vi "nanomsg_ctx_create.vi"(3 "error in":errorcluster) -> (0 "error out":errorcluster, 2 "context out":refnum<class "nanomsg_context.lvclass">)   [LabVIEW 2014, in "nanomsg.lvlib" / "nanomsg_context.lvclass"]
doc: "Instantiate Nanomsg and return a <b>context</b> to create sockets with. Ideally, this should only be called once per application and the context shared."
uses:
  nanomsg_context.lvclass
  nanomsg_context.lvclass/nanomsg_context.ctl
  <vilib>/Utility/error.llb/Error Cluster From Error Code.vi
  nanomsg.lvlib
panel:
  # "NN"
  # "labview"
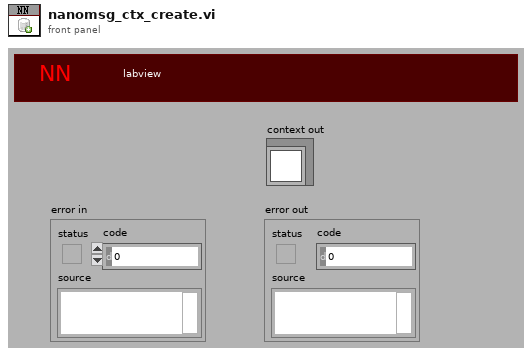
[diagram p1: front panel]
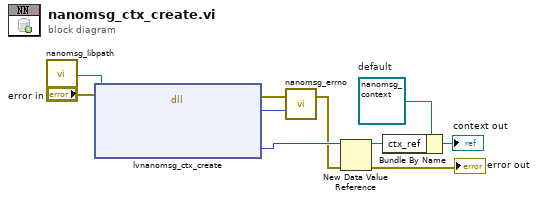
[diagram p0: block diagram]
diagram:
  w9 = refnum<class "nanomsg_context.lvclass"> refnum  # default
  n1 = call "nanomsg_libpath.vi"() -> ("path"=w6:path)
  n2 = dll-call lib="?" fn="lvnanomsg_ctx_create" ("zmq_labview.dll:lvzmq_init")(path in=w6, error in="error in") -> (error out=w5:errorcluster, "return value"=w4:i32, "ctx_obj"=w3:u64)  [unwired: 4 in, 1 out]
  n3 = call "nanomsg_errno.vi"("retval"=w4, "error in"=w5) -> ("error out"=w2:errorcluster)  [unwired: 1 out]
  n4 = New Data Value Reference(data value=w3, error in=w2) -> (data value reference=w1:refnum<data-value>, error out=→"error out":errorcluster)
  n5 = Bundle By Name(cluster=w9, "ctx_ref"=w1) -> (→"context out":refnum<class "nanomsg_context.lvclass">)
